vi "Build ALL.vi"(5 "FP Version":string="4.57.6.7", 7 "TC Version":string="4.61.5.6", 8 "Dry Run?":bool, 9 "FP EXE":bool=TRUE, 10 "TC EXE":bool=TRUE, 11 "Package":bool) -> ()   [LabVIEW 2019]
uses:
  <vilib>/JKI/VIPM API/VIPM API_vipm_api.lvlib
  <vilib>/MakerHub/Toolbox/LMH-Toolbox.lvlib
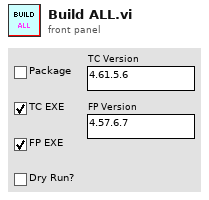
[diagram p1: front panel]
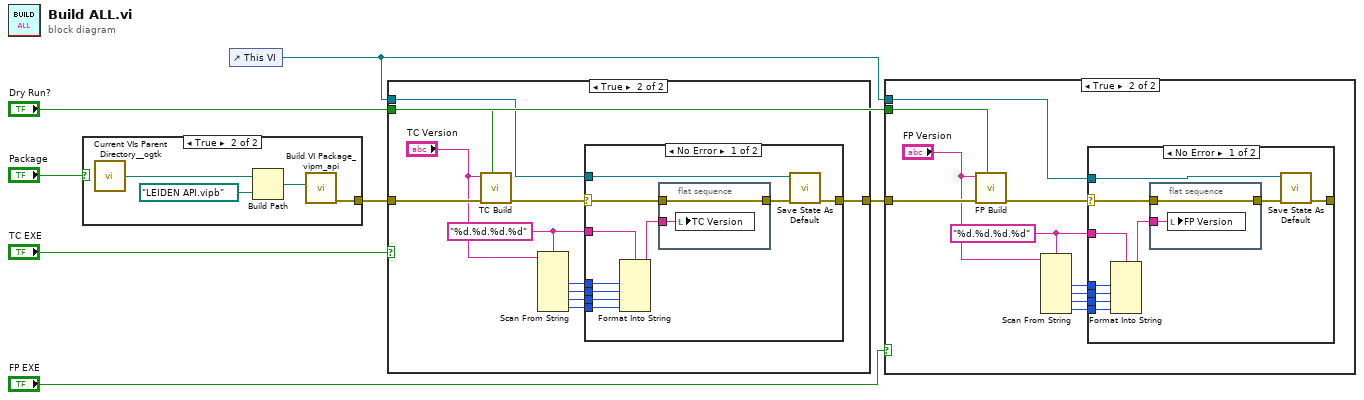
[diagram p0: block diagram]
diagram:
  n1 = case shown="True" "Package" {
    tunnel: [_ w8] -> w6
    frame False {
    }
    frame True {
      n2 = call <userlib>:"Current VIs Parent Directory__ogtk.vi"() -> ("Parent Directory (+ Relative)"=w11:path)  [unwired: 5 in]
      n3 = Build Path(base path=w11, name or relative path=path "LEIDEN API.vipb" ("Path to VIPB File")) -> (appended path=w9:path)
      n4 = call <vilib>:"Build VI Package_vipm_api.vi"("Path to VIPB File"=w9) -> ("error out"=w8:errorcluster)  [unwired: 9 in, 1 out]
    }
  }
  n5 = control-ref of="This VI"() -> (w1:refnum<vi>)
  n6 = case shown="True" "TC EXE" {
    tunnel: [w12 w15] -> w7
    tunnel: w6 -> [w12 w23]
    tunnel: "Dry Run?" -> [_ w22]
    tunnel: w1 -> [_ w13]
    frame False {
    }
    frame True {
      w17 = "%d.%d.%d.%d" ("format string")
      n7 = call "TC Build.vi"("Dry Run?"=w22, "error in"=w23, "Package Version"="TC Version") -> ("Error Out"=w16:errorcluster)  [unwired: 8 in]
      n8 = Scan From String(format string=w17, input string="TC Version") -> (output 1=w18:i32, output 2=w19:i32, output 3=w20:i32, output 4=w21:i32)  [unwired: 6 in, 3 out]
      n9 = case shown="No Error" w16 {
        selector: w16 -> [w25 _]
        tunnel: w13 -> [w33 _]
        tunnel: [w32 _] -> w15
        tunnel: w18 -> [w30 _]
        tunnel: w19 -> [w29 _]
        tunnel: w20 -> [w28 _]
        tunnel: w21 -> [w24 _]
        tunnel: w17 -> [w27 _]
        frame No Error {
          n10 = Format Into String(format string=w27, w30, w29, w28, w24) -> (resulting string=w31:string)  [unwired: 2 in, 1 out]
          n11 = flat-sequence {
            tunnel: w31 -> [w35]
            tunnel: [w34] -> w26
            tunnel: w25 -> [w34]
            frame #0 {
              n12 = local write "TC Version"(w35) -> ()
            }
          }
          n13 = call <vilib>:"Save State As Default.vi"("Error In"=w26, "Target VI"=w33) -> ("Error Out"=w32:errorcluster)  [unwired: 8 in, 1 out]
        }
        frame Error {
        }
      }
    }
  }
  n14 = case shown="True" "FP EXE" {
    tunnel: w7 -> [_ w45]
    tunnel: "Dry Run?" -> [_ w44]
    tunnel: w1 -> [_ w37]
    frame False {
    }
    frame True {
      w43 = "%d.%d.%d.%d" ("format string")
      n15 = call "FP Build.vi"("Dry Run?"=w44, "error in"=w45, "Package Version"="FP Version") -> ("Error Out"=w38:errorcluster)  [unwired: 8 in]
      n16 = Scan From String(format string=w43, input string="FP Version") -> (output 1=w42:i32, output 2=w41:i32, output 3=w40:i32, output 4=w39:i32)  [unwired: 6 in, 3 out]
      n17 = case shown="No Error" w38 {
        selector: w38 -> [w47 _]
        tunnel: w37 -> [w55 _]
        tunnel: [w54 _] -> _
        tunnel: w42 -> [w52 _]
        tunnel: w41 -> [w51 _]
        tunnel: w40 -> [w50 _]
        tunnel: w39 -> [w46 _]
        tunnel: w43 -> [w49 _]
        frame No Error {
          n18 = Format Into String(format string=w49, w52, w51, w50, w46) -> (resulting string=w53:string)  [unwired: 2 in, 1 out]
          n19 = flat-sequence {
            tunnel: w53 -> [w57]
            tunnel: [w56] -> w48
            tunnel: w47 -> [w56]
            frame #0 {
              n20 = local write "FP Version"(w57) -> ()
            }
          }
          n21 = call <vilib>:"Save State As Default.vi"("Error In"=w48, "Target VI"=w55) -> ("Error Out"=w54:errorcluster)  [unwired: 8 in, 1 out]
        }
        frame Error {
        }
      }
    }
  }
